vi "Ejer2_ComparadorDeDatos.vi"() -> ()   [LabVIEW 2020]
panel:
  out "ACCESO PERMITIDO":bool[](array[boolean])
  in  "stop":bool
  in  "CONTRASEÑA DE USUARIOS":string[](array[string])
  in  "USUARIOS":string[](array[string])
  in  "CONTRASEÑA":string
  in  "USUARIO":string
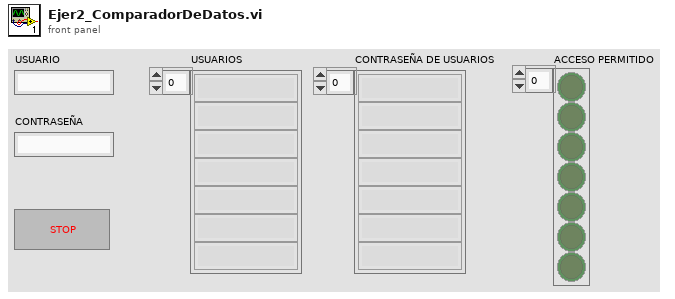
[diagram p1: front panel]
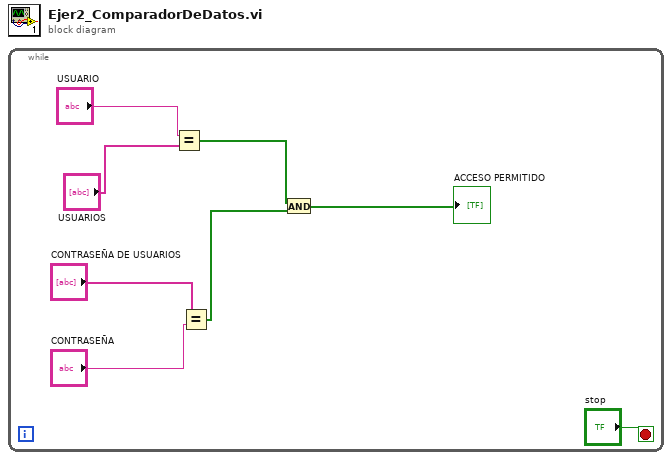
[diagram p0: block diagram]
diagram:
  n1 = while {
    stop <- "stop" stop-if-true
    n2 = Equal?(x="USUARIO", y="USUARIOS") -> (x = y?=w4:bool[])
    n3 = Equal?(x="CONTRASEÑA DE USUARIOS", y="CONTRASEÑA") -> (x = y?=w3:bool[])
    n4 = And(x=w4, y=w3) -> (x .and. y?=→"ACCESO PERMITIDO":bool[])
  }
